vi "Decorate.vi"(10 "Event":refnum<class "Event.lvclass">, 11 "Event in":refnum<class "Event.lvclass">) -> (3 "Event out":refnum<class "Event.lvclass">)   [LabVIEW 2021, in "jettl.lvlib" / "Event.lvclass"]
uses:
  Event.lvclass
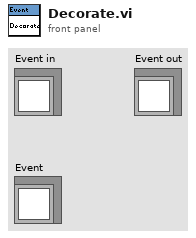
[diagram p1: front panel]
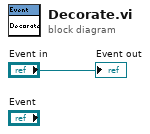
[diagram p0: block diagram]
diagram:
  "Event out" <- "Event in"
